vi "Get Monkey Picture.vi"() -> (0 "Monkey":picture)   [LabVIEW 2020, in "Monkey.lvlib" / "Monkey.lvclass"]
uses:
  Monkey.lvclass
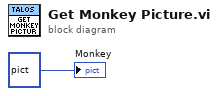
[diagram p0: block diagram]
diagram:
  "Monkey" <- picture bytes[3230] ("Monkey")
